vi "Write Motors with Encoders Class.vi"(8 "error in (no error)":errorcluster, 10 "Motors with Encoders.lvlib:Motors with Encoders.lvclass":refnum<class "Motors with Encoders.lvclass">, 11 "Operator in":refnum<class "Operator.lvclass">) -> (0 "error out":errorcluster, 3 "Operator out":refnum<class "Operator.lvclass">)   [LabVIEW 2014, in "Operator.lvlib" / "Operator.lvclass"]
uses:
  Operator.lvclass
  Motor with Encoders/Motors with Encoders Class/Motors with Encoders.lvclass
  Operator.lvclass/Operator.ctl
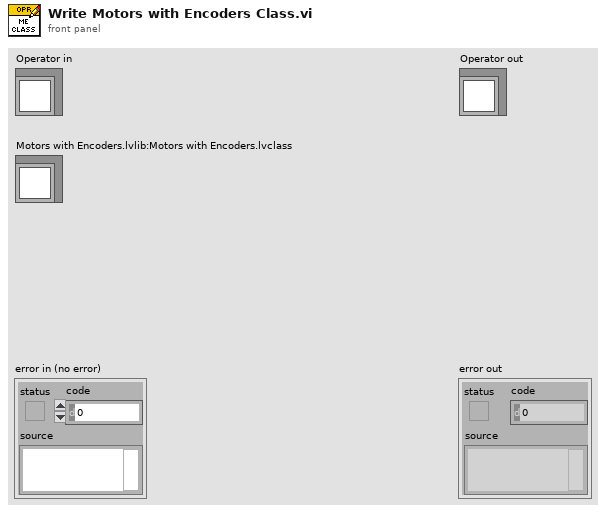
[diagram p1: front panel]
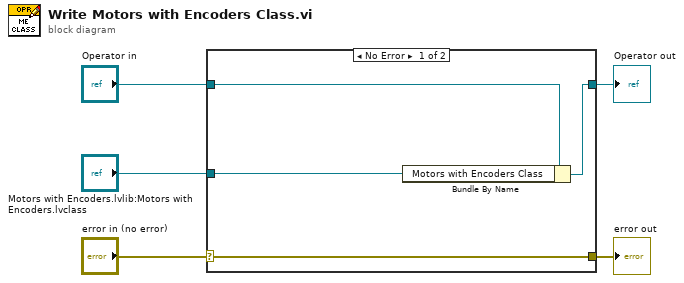
[diagram p0: block diagram]
diagram:
  n1 = case shown="No Error" "error in (no error)" {
    selector: "error in (no error)" -> [w9 w10]
    tunnel: [w9 w10] -> w4
    tunnel: [w7 w11] -> w2
    tunnel: "Operator in" -> [w8 w11]
    tunnel: "Motors with Encoders.lvlib:Motors with Encoders.lvclass" -> [w6 _]
    frame No Error {
      n2 = Bundle By Name(cluster=w8, "Motors with Encoders Class"=w6) -> (w7:refnum<class "Operator.lvclass">)
    }
    frame Error {
    }
  }
  "error out" <- w4
  "Operator out" <- w2
